vi "Set Icon.vi"(0 "VI":refnum<vi>, 5 "user-supplied text (\"\" - use VI file name)":string, 11 "error in":errorcluster) -> (4 "Error Message":string, 15 "error out":errorcluster)   [LabVIEW 2020, in "Text-Based VI Icon.lvlib"]
uses:
  <vilib>/LabVIEW Icon API/Set Text Icon/Text-Based VI Icon.lvlib
  <vilib>/LabVIEW Icon API/Set Text Icon/Library Icon Information.ctl
  <vilib>/LabVIEW Icon API/Set Text Icon/User Visible Strings.vi
  <vilib>/LabVIEW Icon API/lv_icon/Classes/Icon/Icon.lvclass
  <vilib>/LabVIEW Icon API/LabVIEW Icon API.lvlib
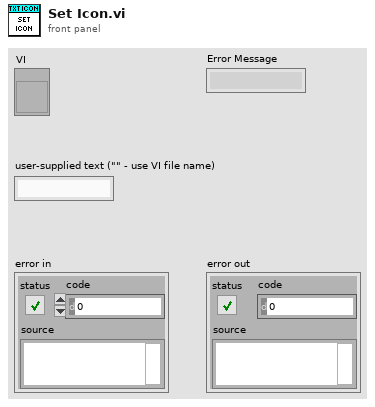
[diagram p1: front panel]
types:
  T1 = typedef "Text-Based VI Icon.lvlib/Library Icon Information.ctl" = cluster{"Library Path":path, "Number of Pixel Rows in Icon":i32, "Icon Image":picture}
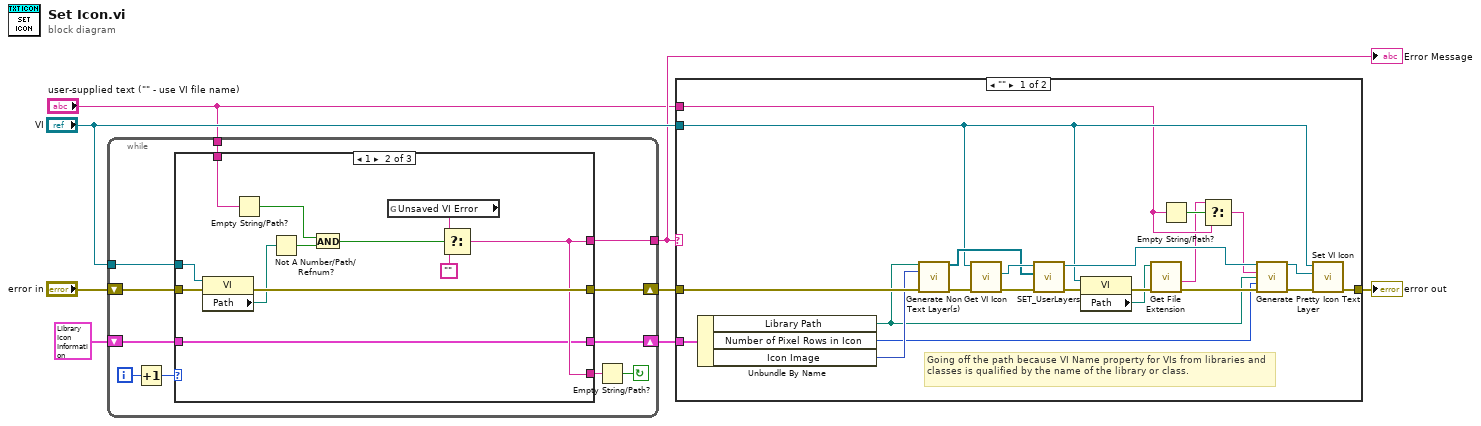
[diagram p0: block diagram]
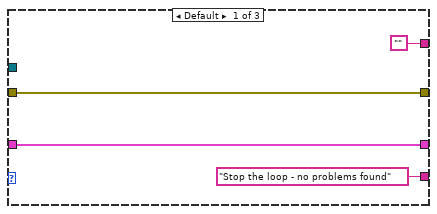
[diagram p3: hidden frame]
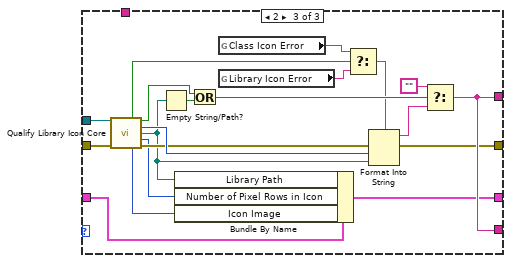
[diagram p4: hidden frame]
diagram:
  n1 = while {
    tunnel: "VI" -> [w17]
    shift-right: [w18] -> w6
    shift-left: "error in" -> [w19]
    tunnel: [w14] -> w4
    shift-right: [w10] -> w2
    shift-left: T1 {"Library Path"=path "", "Number of Pixel Rows in Icon"=0, "Icon Image"=bytes[0]} ("Library Icon Information") -> [w11]
    tunnel: "user-supplied text (\"\" - use VI file name)" -> [w9]
    i -> [w15]
    stop <- w13 continue-if-true
    n2 = Increment(x=w15) -> (x+1=w16:i32)
    n3 = case shown="1" w16 {
      tunnel: w19 -> [w23 w35 w53]
      tunnel: [w23 w34 w45] -> w18
      tunnel: w17 -> [_ w33 w54]
      tunnel: ["" w29 w55] -> w14
      tunnel: ["Stop the loop - no problems found" w29 w55] -> w12
      tunnel: w11 -> [w20 w27 w39]
      tunnel: [w20 w27 w38] -> w10
      tunnel: w9 -> [_ w26 _]
      frame Default {
      }
      frame 1 {
        n4 = property class="VI"(reference=w33, error in=w35) -> (error out=w34:errorcluster, "Path"=w32:path)  [unwired: 1 out]
        n5 = Empty String/Path?(string/path=w26) -> (empty?=w24:bool)
        n6 = Not A Number/Path/Refnum?(number/path/refnum=w32) -> (NaN/Path/Refnum?=w31:bool)
        n7 = And(x=w24, y=w31) -> (x .and. y?=w25:bool)
        n8 = global read "User Visible Strings.vi" "Unsaved VI Error"() -> (w28:string)
        n9 = Select(t=w28, s=w25, f="") -> (s? t:f=w29:string)
      }
      frame 2 {
        n10 = call <vilib>:"Qualify Library Icon Core.vi"("VI Reference"=w54, "error in"=w53) -> ("Class?"=w43:bool, "Good Library Icon"=w52:bool, "Maximum Number of Rows"=w47:i32, "Library Path"=w40:path, "Number of Rows in Icon"=w37:i32, "Icon Image"=w36:picture, "error out"=w46:errorcluster)  [unwired: 7 in]
        n11 = Empty String/Path?(string/path=w40) -> (empty?=w48:bool)
        n12 = Bundle By Name(cluster=w39, "Library Path"=w40, "Number of Pixel Rows in Icon"=w37, "Icon Image"=w36) -> (w38:T1)
        n13 = Or(x=w52, y=w48) -> (x .or. y?=w50:bool)
        n14 = global read "User Visible Strings.vi" "Class Icon Error"() -> (w41:string)
        n15 = global read "User Visible Strings.vi" "Library Icon Error"() -> (w42:string)
        n16 = Select(t=w41, s=w43, f=w42) -> (s? t:f=w44:string)
        n17 = Format Into String(format string=w44, error in=w46, w47, w40) -> (resulting string=w49:string, error out=w45:errorcluster)  [unwired: 1 in]
        n18 = Select(t="", s=w50, f=w49) -> (s? t:f=w55:string)
      }
    }
    n19 = Empty String/Path?(string/path=w12) -> (empty?=w13:bool)
  }
  "Error Message" <- w4
  n20 = case shown="\"\"" w4 {
    tunnel: [w77 w78] -> w8
    tunnel: w6 -> [w68 w78]
    tunnel: "VI" -> [w64 _]
    tunnel: w2 -> [w63 _]
    tunnel: "user-supplied text (\"\" - use VI file name)" -> [w58 _]
    frame "" {
      # "Going off the path because VI Name property for VIs from libraries and classes is qualified by the name of the library or class."
      n21 = Unbundle By Name(w63) -> ("Library Path"=w61:path, "Number of Pixel Rows in Icon"=w60:i32, "Icon Image"=w62:picture)
      n22 = call <vilib>:"Generate Non Text Layer(s).vi"("Library Path"=w61, "new picture"=w62, "error in"=w68) -> ("Layers"=w72:refnum<class "Layer.lvclass">[], "error out"=w74:errorcluster)  [unwired: 11 in]
      n23 = call <vilib>:"Get VI Icon.vi"("error in (no error)"=w74, "VI Refnum in"=w64) -> ("error out"=w75:errorcluster, "Icon"=w76:refnum<class "Icon.lvclass">)  [unwired: 7 in, 1 out]
      n24 = call-dynamic "SET_UserLayers.vi"("error in (no error)"=w75, "Layers"=w72, "Icon.lvclass in"=w76) -> ("error out"=w67:errorcluster, "Icon.lvclass out"=w73:refnum<class "Icon.lvclass">)  [unwired: 7 in]
      n25 = property class="VI"(reference=w64, error in=w67) -> (error out=w66:errorcluster, "Path"=w65:path)  [unwired: 1 out]
      n26 = call <vilib>:"Get File Extension.vi"("error in (no error)"=w66, "file"=w65) -> ("error out"=w71:errorcluster, "filename without extension"=w56:string)  [unwired: 5 in, 3 out]
      n27 = Empty String/Path?(string/path=w58) -> (empty?=w59:bool)
      n28 = Select(t=w56, s=w59, f=w58) -> (s? t:f=w57:string)
      n29 = call <vilib>:"Generate Pretty Icon Text Layer.vi"("Icon in"=w73, "VI Name"=w57, "Library Path"=w61, "Number of Rows in Icon"=w60, "error in (no error)"=w71) -> ("Icon out"=w69:refnum<class "Icon.lvclass">, "error out"=w70:errorcluster)  [unwired: 9 in]
      n30 = call <vilib>:"Set VI Icon.vi"("error in (no error)"=w70, "Icon"=w69, "VI Refnum in"=w64) -> ("error out"=w77:errorcluster)  [unwired: 7 in, 1 out]
    }
    frame Default {
    }
  }
  "error out" <- w8
